vi "Generate_WayPoints_Hopping_runningAverage.vi"(8 "element":u16=8, 11 "Input Cluster":T2={"Scan Rate (um/s)"=15.0, "X Start"=15.0, "X End"=15.0, "Y Start"=15.0, "Y End"=15.0, " Z Start"=15.0, "HoppingDistance"=1.0, "V"=15.0, "Z End"=15.0, "Approach Rate Hopping (um/s)"=15.0, "Retrack Rate (um/s)"=15.0, "V 2"=15.0, "Approach Rate (um/s)"=15.0, "Hold Time START / s"=15.0, "Hold Time Delta / s"=15.0, "Voltage to Electrode During Retract"=0.0, "Pause on First Approach?"=FALSE}) -> (1 "output cluster":T1)   [LabVIEW 2023]
uses:
  TypeDefs/WayPointCluster.ctl
panel:
  in  "WayPointCluster":T1
  out "Y  P":dbl
  out "X  P":dbl
  out "HoppingDistanceX":dbl
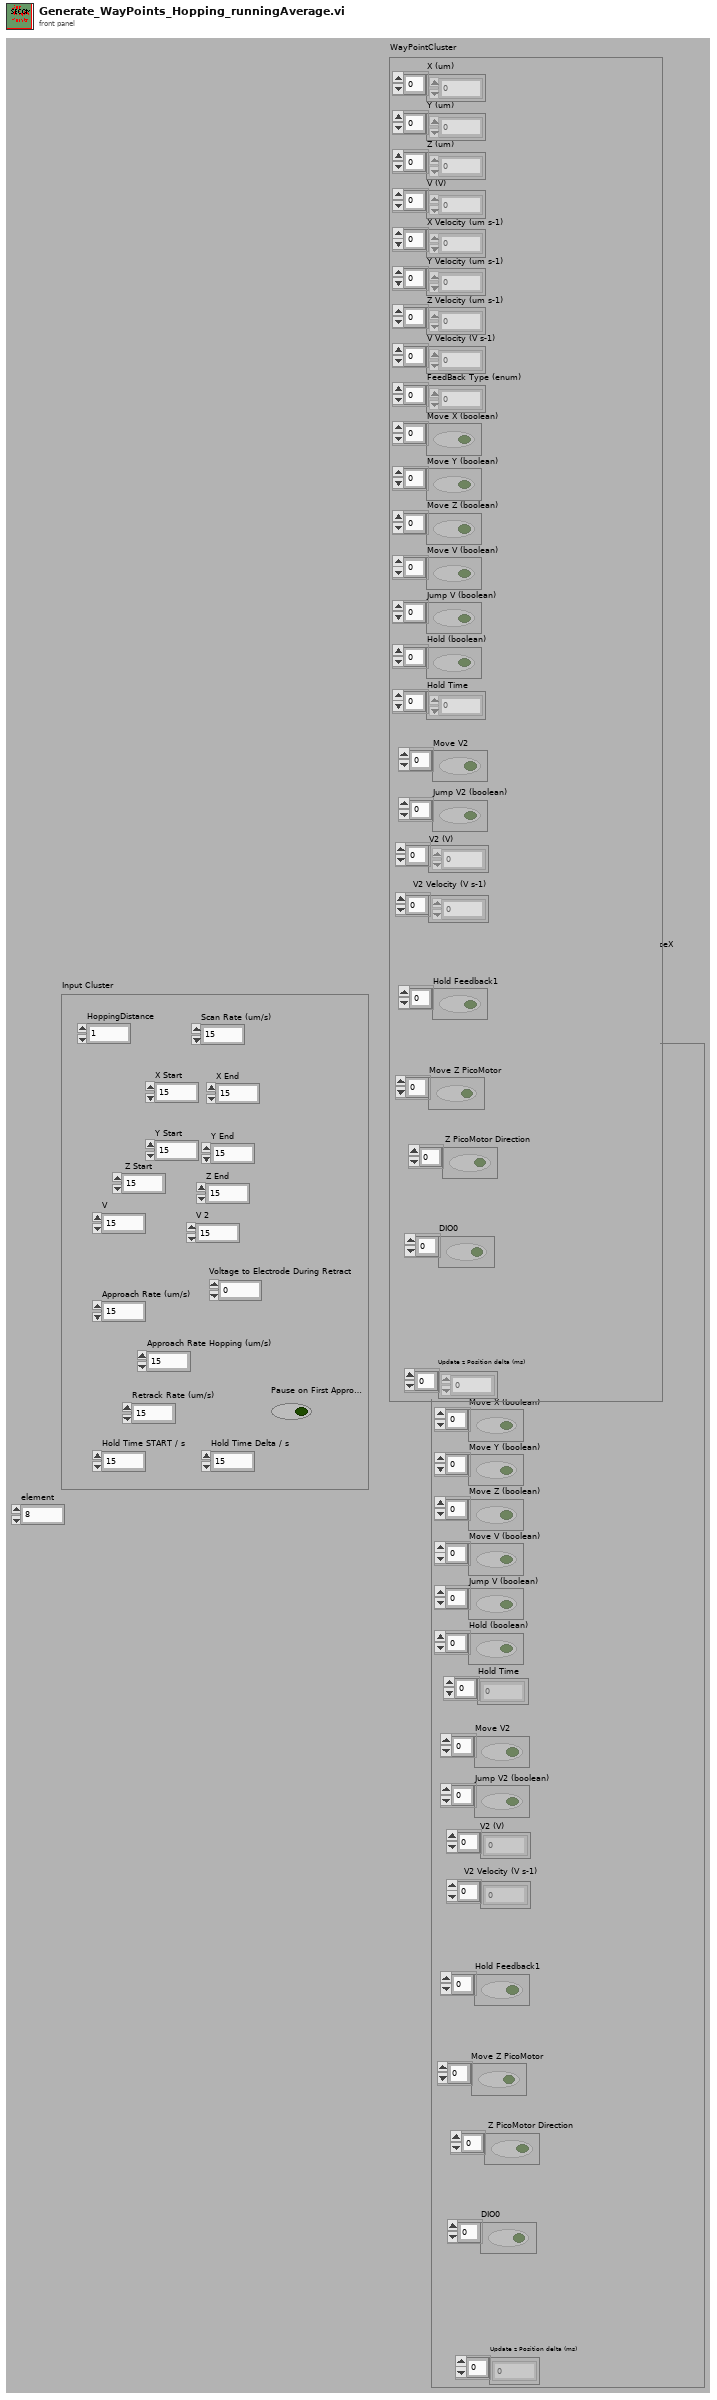
[diagram p1: front panel]
types:
  T1 = typedef "WayPointCluster.ctl" = cluster{"X (um)":dbl[], "Y (um)":dbl[], "Z (um)":dbl[], "V (V)":dbl[], "X Velocity (um s-1)":dbl[], "Y Velocity (um s-1)":dbl[], "Z Velocity (um s-1)":dbl[], "V Velocity (V s-1)":dbl[], "FeedBack Type (enum)":u16[], "Move X (boolean)":bool[], "Move Y (boolean)":bool[], "Move Z (boolean)":bool[], "Move V (boolean)":bool[], "Jump V (boolean)":bool[], "Hold (boolean)":bool[], "Hold Time":u32[], "V2 (V)":dbl[], "Move V2":bool[], "V2 Velocity (V s-1)":dbl[], "Jump V2 (boolean)":bool[], "Update z Position delta (ms)":i16[], "Hold Feedback1":bool[], "Move Z PicoMotor":bool[], " Z PicoMotor Direction":bool[], "DIO0":bool[]}
  T2 = cluster{"Scan Rate (um/s)":dbl, "X Start":dbl, "X End":dbl, "Y Start":dbl, "Y End":dbl, " Z Start":dbl, "HoppingDistance":dbl, "V":dbl, "Z End":dbl, "Approach Rate Hopping (um/s)":dbl, "Retrack Rate (um/s)":dbl, "V 2":dbl, "Approach Rate (um/s)":dbl, "Hold Time START / s":dbl, "Hold Time Delta / s":dbl, "Voltage to Electrode During Retract":dbl, "Pause on First Approach?":bool}
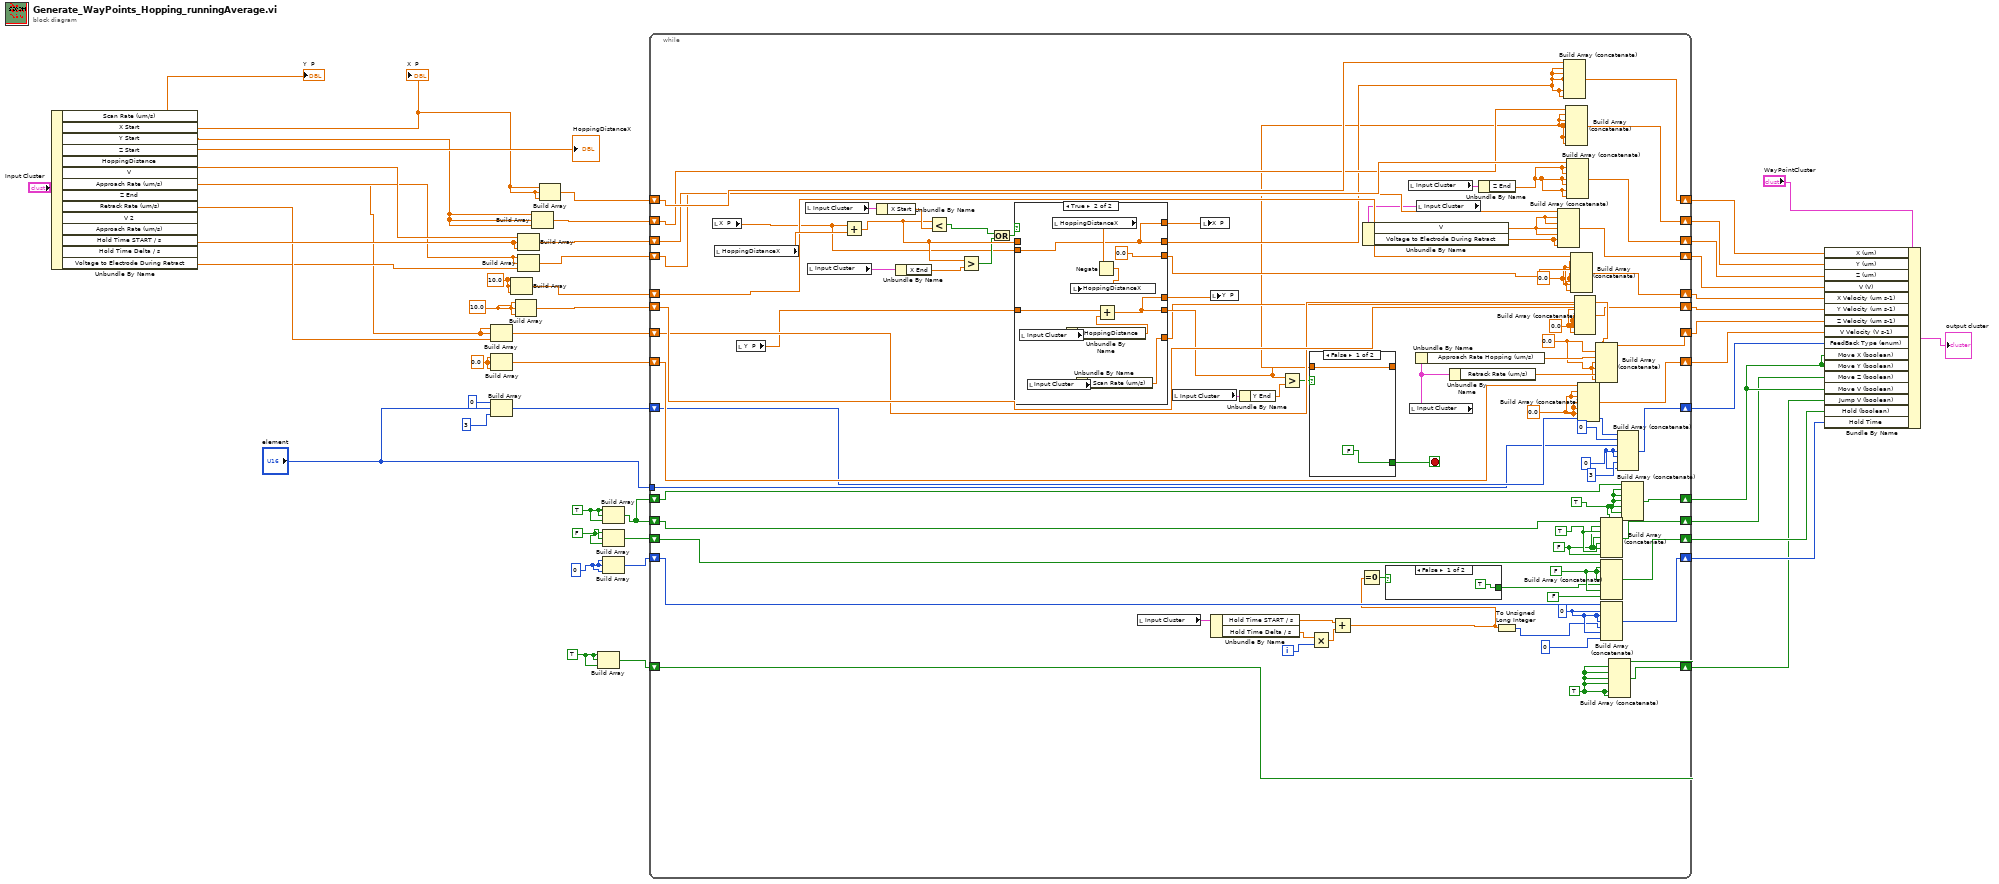
[diagram p0: block diagram]
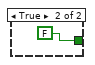
[diagram p2: hidden frame]
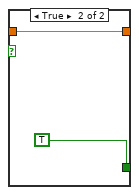
[diagram p3: hidden frame]
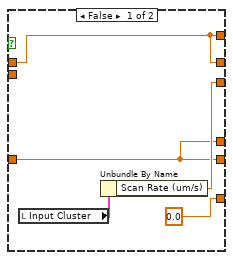
[diagram p4: hidden frame]
diagram:
  w10 = TRUE
  w11 = u32 0 ("element")
  w12 = FALSE
  w13 = TRUE
  w6 = 10.0 ("element")
  w7 = 10.0 ("element")
  w9 = 0.0 ("element")
  n1 = Unbundle By Name("Input Cluster") -> ("X Start"=w29:dbl, "Y Start"=w28:dbl, "Z Start"=w30:dbl, "HoppingDistance"=→"HoppingDistanceX":dbl, "V"=w26:dbl, "Approach Rate (um/s)"=w8:dbl, "Z End"=w27:dbl, "Retrack Rate (um/s)"=w25:dbl, "Voltage to Electrode During Retract"=w15:dbl)  [unwired: 5 out]
  "X  P" <- w29
  "Y  P" <- w28
  n2 = Build Array(w8, w8, w25) -> (w37:dbl[])
  n3 = Build Array(u16 0 ("element"), "element", u16 3 ("element")) -> (w33:u16[])
  n4 = Build Array(w9, w9, w9) -> (w35:dbl[])
  n5 = Build Array(w6, w6, w6) -> (w40:dbl[])
  n6 = Build Array(w7, w7, w7) -> (w39:dbl[])
  n7 = Build Array(w26, w26, w15) -> (w42:dbl[])
  n8 = Build Array(w30, w27, w27) -> (w44:dbl[])
  n9 = Build Array(w28, w28, w28) -> (w46:dbl[])
  n10 = Build Array(w29, w29, w29) -> (w48:dbl[])
  n11 = Build Array(w10, w10, w10) -> (w18:bool[])
  n12 = Build Array(w13, w13, w13) -> (w16:bool[])
  n13 = Build Array(w12, w12, w12) -> (w22:bool[])
  n14 = Build Array(w11, w11, w11) -> (w21:u32[])
  n15 = while {
    shift-right: [w128] -> w47
    shift-left: w48 -> [w129]
    shift-right: [w120] -> w45
    shift-left: w46 -> [w110]
    shift-right: [w119] -> w43
    shift-left: w44 -> [w127]
    shift-right: [w118] -> w41
    shift-left: w42 -> [w126]
    shift-right: [w117] -> w23
    shift-left: w40 -> [w125]
    shift-right: [w116] -> w38
    shift-left: w39 -> [w124]
    shift-right: [w115] -> w36
    shift-left: w37 -> [w123]
    shift-right: [w114] -> w34
    shift-left: w35 -> [w122]
    shift-right: [w113] -> w32
    shift-left: w33 -> [w121]
    shift-right: [w84] -> w2
    shift-left: w16 -> [w83]
    shift-right: [w85] -> w20
    shift-left: w22 -> [w89]
    shift-right: [w86] -> w19
    shift-left: w21 -> [w88]
    shift-right: [w81] -> w17
    shift-left: w18 -> [w82]
    shift-right: [w76] -> w3
    shift-left: w16 -> [w77]
    tunnel: "element" -> [w50]
    i -> [w78]
    stop <- w100 stop-if-true
    w57 = TRUE
    w53 = TRUE
    w70 = u32 0 ("element")
    w71 = FALSE
    w56 = FALSE
    w72 = TRUE
    w58 = u16 0 ("element")
    w61 = 0.0 ("element")
    w62 = 0.0 ("element")
    w59 = 0.0 ("element")
    w60 = 0.0 ("element")
    n16 = local read "X  P"() -> (w98:dbl)
    n17 = local read "HoppingDistanceX"() -> (w130:dbl)
    n18 = local read "Y  P"() -> (w97:dbl)
    n19 = local read "Input Cluster"() -> (w132:T2)
    n20 = local read "Input Cluster"() -> (w131:T2)
    n21 = Add(x=w98, y=w130) -> (x+y=w106:dbl)
    n22 = Unbundle By Name(w132) -> ("X Start"=w109:dbl)
    n23 = Unbundle By Name(w131) -> ("X End"=w107:dbl)
    n24 = Less?(x=w106, y=w109) -> (x < y?=w108:bool)
    n25 = Greater?(x=w106, y=w107) -> (0:w105:bool)
    n26 = Or(x=w108, y=w105) -> (x .or. y?=w104:bool)
    n27 = case shown="True" w104 {
      tunnel: w106 -> [w139 _]
      tunnel: [w139 w145] -> w66
      tunnel: w98 -> [_ w145]
      tunnel: w97 -> [w140 w146]
      tunnel: [w140 w144] -> w96
      tunnel: [w142 0.0] -> w91
      tunnel: [0.0 w147] -> w90
      tunnel: [w140 w144] -> w95
      tunnel: [w139 w145] -> w94
      frame False {
        n28 = local read "Input Cluster"() -> (w143:T2)
        n29 = Unbundle By Name(w143) -> ("Scan Rate (um/s)"=w142:dbl)
      }
      frame True {
        n30 = local read "Input Cluster"() -> (w151:T2)
        n31 = local read "Input Cluster"() -> (w149:T2)
        n32 = local read "HoppingDistanceX"() -> (w153:dbl)
        n33 = Unbundle By Name(w151) -> ("HoppingDistance"=w150:dbl)
        n34 = Unbundle By Name(w149) -> ("Scan Rate (um/s)"=w147:dbl)
        n35 = Negate(x=w153) -> (-x=w152:dbl)
        n36 = local write "HoppingDistanceX"(w152) -> ()
        n37 = Add(x=w146, y=w150) -> (x+y=w144:dbl)
      }
    }
    n38 = local read "Input Cluster"() -> (w87:T2)
    n39 = local read "Input Cluster"() -> (w103:T2)
    n40 = local write "X  P"(w94) -> ()
    n41 = local write "Y  P"(w95) -> ()
    n42 = Unbundle By Name(w87) -> ("Hold Time START / s"=w67:dbl, "Hold Time Delta / s"=w80:dbl)
    n43 = Unbundle By Name(w103) -> ("Y End"=w102:dbl)
    n44 = Greater?(x=w96, y=w102) -> (0:w101:bool)
    n45 = case shown="False" w101 {
      tunnel: w96 -> [w136 w138]
      tunnel: [w136 w138] -> w65
      tunnel: [FALSE TRUE] -> w100
      frame False {
      }
      frame True {
      }
    }
    n46 = Multiply(x=w80, y=w78) -> (x*y=w79:dbl)
    n47 = Add(x=w67, y=w79) -> (x+y=w52:dbl)
    n48 = Equal To 0?(x=w52) -> (x = 0?=w68:bool)
    n49 = case shown="False" w68 {
      tunnel: [TRUE FALSE] -> w69
      frame False {
      }
      frame True {
      }
    }
    n50 = local read "Input Cluster"() -> (w112:T2)
    n51 = local read "Input Cluster"() -> (w99:T2)
    n52 = Unbundle By Name(w99) -> ("Approach Rate Hopping (um/s)"=w92:dbl)
    n53 = local read "Input Cluster"() -> (w111:T2)
    n54 = Unbundle By Name(w111) -> ("V"=w75:dbl, "Voltage to Electrode During Retract"=w63:dbl)
    n55 = Unbundle By Name(w99) -> ("Retrack Rate (um/s)"=w74:dbl)
    n56 = Unbundle By Name(w112) -> ("Z End"=w64:dbl)
    n57 = To Unsigned Long Integer(number=w52) -> (unsigned 32bit integer=w51:u32)
    n58 = Build Array (concatenate)(w126, w75, w75, w75, w75, w63, w63) -> (w118:dbl[])
    n59 = Build Array (concatenate)(w129, w66, w66, w66, w66, w66, w66) -> (w128:dbl[])
    n60 = Build Array (concatenate)(w110, w65, w65, w65, w65, w65, w65) -> (w120:dbl[])
    n61 = Build Array (concatenate)(w127, w64, w64, w64, w64, w64, w64) -> (w119:dbl[])
    n62 = Build Array (concatenate)(w125, w91, w62, w62, w62, w62, w62) -> (w117:dbl[])
    n63 = Build Array (concatenate)(w124, w90, w61, w61, w61, w61, w61) -> (w116:dbl[])
    n64 = Build Array (concatenate)(w122, w59, w59, w59, w59, w59, w59) -> (w114:dbl[])
    n65 = Build Array (concatenate)(w123, w60, w92, w60, w60, w74, w60) -> (w115:dbl[])
    n66 = Build Array (concatenate)(w83, w56, w72, w56, w56, w72, w56) -> (w84:bool[])
    n67 = Build Array (concatenate)(w89, w71, w71, w71, w69, w71, FALSE ("element")) -> (w85:bool[])
    n68 = Build Array (concatenate)(w88, w70, w70, w70, w51, w70, u32 0 ("element")) -> (w86:u32[])
    n69 = Build Array (concatenate)(w82, w53, w53, w53, w53, w53, w53) -> (w81:bool[])
    n70 = Build Array (concatenate)(w121, u16 0 ("element"), w50, w58, w58, u16 3 ("element"), w58) -> (w113:u16[])
    n71 = Build Array (concatenate)(w77, w57, w57, w57, w57, w57, w57) -> (w76:bool[])
  }
  n72 = Bundle By Name(cluster="WayPointCluster", "X (um)"=w47, "Y (um)"=w45, "Z (um)"=w43, "V (V)"=w41, "X Velocity (um s-1)"=w23, "Y Velocity (um s-1)"=w38, "Z Velocity (um s-1)"=w36, "V Velocity (V s-1)"=w34, "FeedBack Type (enum)"=w32, "Move X (boolean)"=w3, "Move Y (boolean)"=w3, "Move Z (boolean)"=w2, "Move V (boolean)"=w3, "Jump V (boolean)"=w17, "Hold (boolean)"=w20, "Hold Time"=w19) -> (→"output cluster":T1)
